vi "Render.vi"(8 "error in":errorcluster, 10 "Renderer in":refnum<class "Renderer.lvclass">, 11 "Custom Errors in":refnum<class "Custom Errors.lvclass">) -> (0 "error out":errorcluster, 3 "Sections out":refnum<class "Section.lvclass">[](array[class]))   [LabVIEW 2021, in "TAF Proj Document Type.lvlib" / "Custom Errors.lvclass"]
uses:
  <vilib>/Wovalab/AntiDoc/Document Type/Add-ons/LabVIEW TAF Project/Custom Errors/Custom Errors.lvclass
  C:/Program Files (x86)/National Instruments/LabVIEW 2021/vi.lib/Wovalab/AntiDoc/Bloc/Bloc.lvclass
  <vilib>/Wovalab/AsciiDoc for LabVIEW/Section/Section.lvclass
  <vilib>/Wovalab/AntiDoc/Renderer/Renderer.lvclass
  <vilib>/Wovalab/AsciiDoc for LabVIEW/Admonition/Types--enum.ctl
  <vilib>/Wovalab/AsciiDoc for LabVIEW/Table/Column Attributes--cluster.ctl
  <vilib>/Wovalab/AsciiDoc for LabVIEW/Table/Horizontal Alignment--enum.ctl
  <vilib>/Wovalab/AsciiDoc for LabVIEW/Table/Vertical Alignment--enum.ctl
  <vilib>/Wovalab/AsciiDoc for LabVIEW/Table/Style--enum.ctl
  <vilib>/Wovalab/AntiDoc/Bloc/Bloc.lvclass/Bloc.ctl
  <vilib>/Wovalab/AsciiDoc for LabVIEW/Table/Table.lvclass/Table.ctl
  <vilib>/Wovalab/AntiDoc/Bloc/Read Name.vi
  <vilib>/Wovalab/AsciiDoc for LabVIEW/Admonition/Admonition.lvclass
  C:/Program Files (x86)/National Instruments/LabVIEW 2021/vi.lib/Wovalab/AsciiDoc for LabVIEW/Adoc-Bloc/Bloc.lvclass
  <vilib>/Wovalab/AsciiDoc for LabVIEW/Table/Table.lvclass
  <vilib>/Wovalab/AsciiDoc for LabVIEW/Section/Add Bloc (array).vi
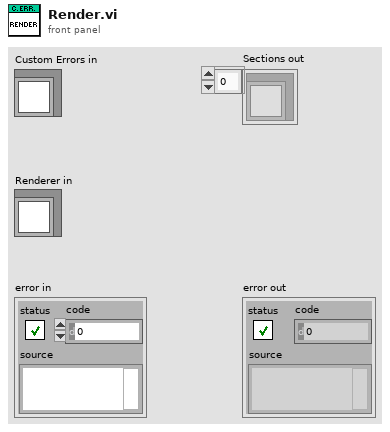
[diagram p1: front panel]
types:
  T1 = typedef "Wovalab_lib_AsciiDoctor.lvlib/Table.lvclass/Column Attributes--cluster.ctl" = cluster{"Width":u16, "Horizontal Alignment":T2, "Vertical Alignment":T3, "Style":T4}
  T2 = typedef "Wovalab_lib_AsciiDoctor.lvlib/Table.lvclass/Horizontal Alignment--enum.ctl" = enum16{"Left", "Center", "Right"}
  T3 = typedef "Wovalab_lib_AsciiDoctor.lvlib/Table.lvclass/Vertical Alignment--enum.ctl" = enum16{"Top", "Middle", "Bottom"}
  T4 = typedef "Wovalab_lib_AsciiDoctor.lvlib/Table.lvclass/Style--enum.ctl" = enum16{"None", "AsciiDoc", "Emphasis", "Header", "Literal", "Monospaced", "Strong", "Verse"}
  T5 = typedef "Wovalab_lib_AsciiDoctor.lvlib/Admonition.lvclass/Types--enum.ctl" = enum16{"Note", "Tip", "Important", "Warning", "Caution"}
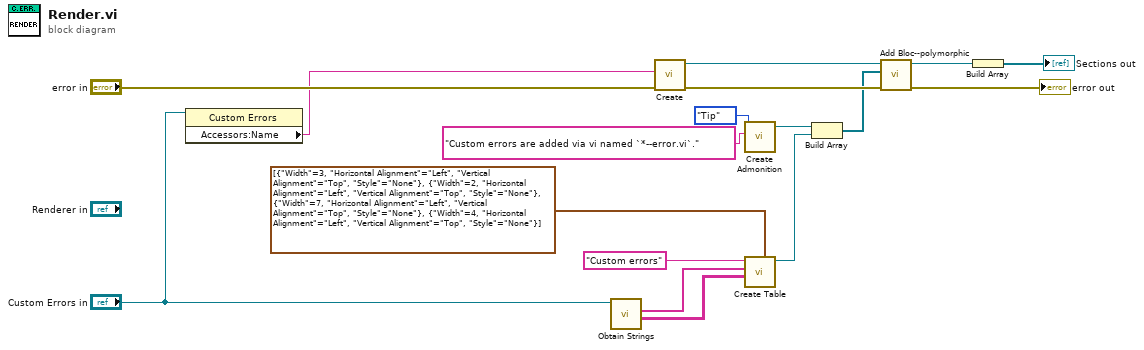
[diagram p0: block diagram]
diagram:
  n1 = property class="Custom Errors"(reference="Custom Errors in") -> ("Accessors:Name"=w3:string)  [unwired: 1 in, 2 out]
  n2 = call <vilib>:"Obtain Strings.vi"("Custom Errors in"="Custom Errors in") -> ("Strings"=w6:string[][], "Header"=w7:string[])  [unwired: 7 in, 2 out]
  n3 = call <vilib>:"Create.vi"("error in (no error)"="error in", "Title"=w3) -> ("error out"=w16:errorcluster, "Section out"=w9:refnum<class "Section.lvclass">)  [unwired: 8 in]
  n4 = call <vilib>:"Create Admonition.vi"("Content"="Custom errors are added via vi named `*--error.vi`.", "Types"=Types--enum."Tip") -> ("Admonition out"=w10:refnum<class "Admonition.lvclass">)  [unwired: 8 in, 1 out]
  n5 = call <vilib>:"Create Table.vi"("Column Attributes"=T1[] [{"Width"=3, "Horizontal Alignment"=enum."Left", "Vertical Alignment"=enum."Top", "Style"=enum."None"}, {"Width"=2, "Horizontal Alignment"=enum."Left", "Vertical Alignment"=enum."Top", "Style"=enum."None"}, {"Width"=7, "Horizontal Alignment"=enum."Left", "Vertical Alignment"=enum."Top", "Style"=enum."None"}, {"Width"=4, "Horizontal Alignment"=enum."Left", "Vertical Alignment"=enum."Top", "Style"=enum."None"}], "Content"=w6, "Header"=w7, "Title"="Custom errors") -> ("Table out"=w13:refnum<class "Table.lvclass">)  [unwired: 6 in, 1 out]
  n6 = Build Array(w10, w13) -> (w8:refnum<class "Bloc.lvclass">[])
  n7 = call-poly <vilib>:"Add Bloc--polymorphic.vi"("error in"=w16, "Bloc"=w8, "Section in"=w9) -> ("error out"=→"error out":errorcluster, "Section out"=w2:refnum<class "Section.lvclass">)  [unwired: 7 in]
  n8 = Build Array(w2) -> (→"Sections out":refnum<class "Section.lvclass">[])
